vi "get_external_stop_v2.vi"(8 "ref_stop_internal":refnum<vi>, 11 "ref_stop_external":refnum<vi>) -> (3 "stop_output":bool)   [LabVIEW 2019]
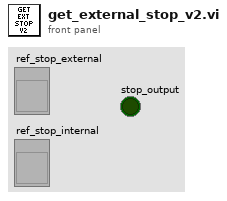
[diagram p1: front panel]
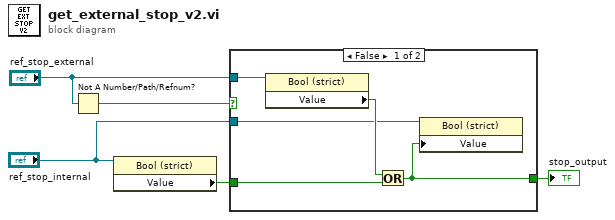
[diagram p0: block diagram]
diagram:
  n1 = Not A Number/Path/Refnum?(number/path/refnum="ref_stop_external") -> (NaN/Path/Refnum?=w4:bool)
  n2 = property on="Property Node" class="Bool (strict)"(reference="ref_stop_internal") -> ("Value"=w3:bool)  [unwired: 1 in, 2 out]
  n3 = case shown="False" w4 {
    tunnel: [w7 w11] -> w2
    tunnel: "ref_stop_external" -> [w10 _]
    tunnel: w3 -> [w9 w11]
    tunnel: "ref_stop_internal" -> [w6 _]
    frame False {
      n4 = property class="Bool (strict)"(reference=w10) -> ("Value"=w8:bool)  [unwired: 1 in, 2 out]
      n5 = Or(x=w8, y=w9) -> (x .or. y?=w7:bool)
      n6 = property on="Property Node" class="Bool (strict)"(reference=w6, "Value"=w7) -> ()  [unwired: 1 in, 2 out]
    }
    frame True {
    }
  }
  "stop_output" <- w2
